vi "SectionA04_Week5_Stus_Subvi.vi"(9 "Frequency of Input (mHz)":dbl, 10 "Gain":dbl, 11 "Peak Voltage of Input":dbl) -> (3 "Array":dbl[][](array[numeric]))   [LabVIEW 2013]
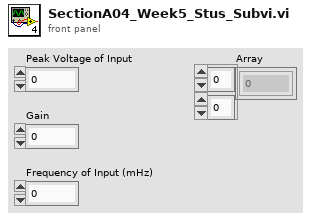
[diagram p1: front panel]
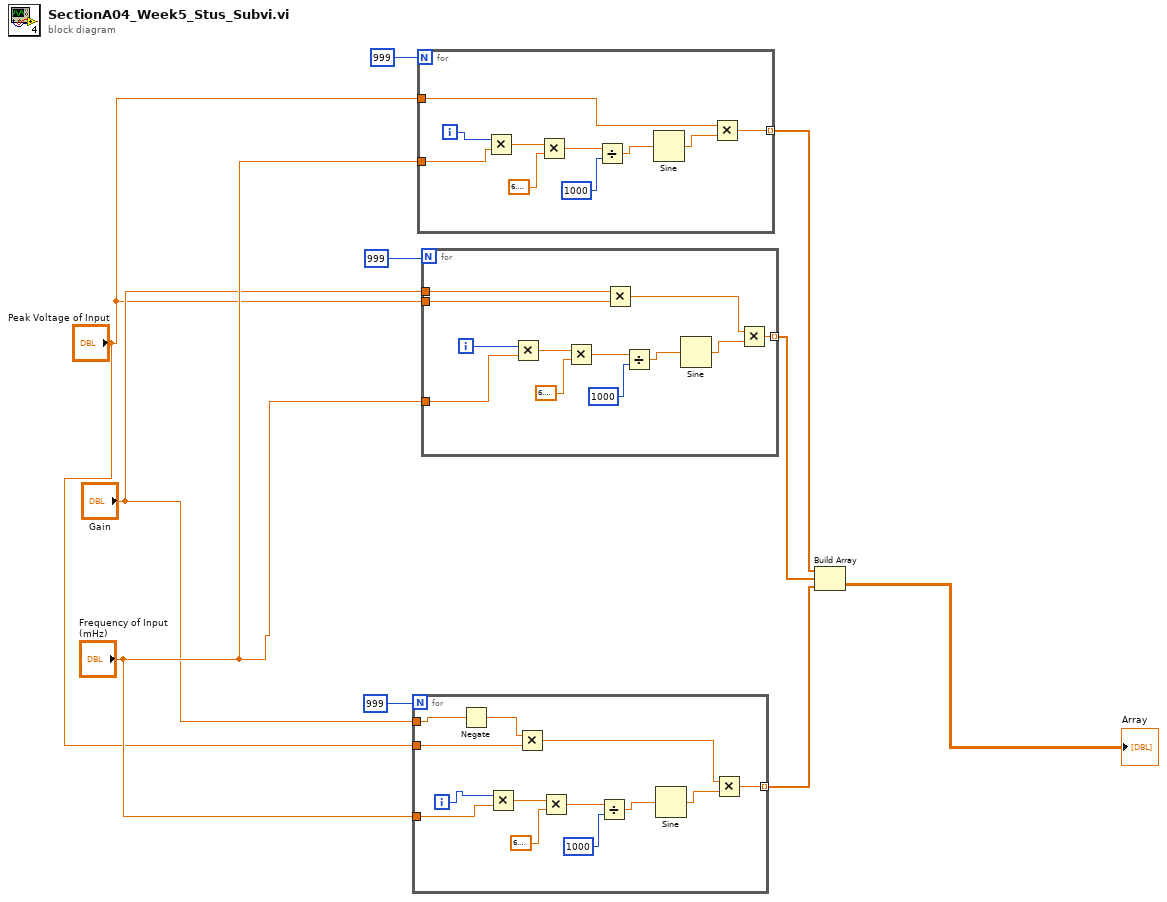
[diagram p0: block diagram]
diagram:
  n1 = for {
    N: 999 -> [_]
    tunnel: "Frequency of Input (mHz)" -> [w17]
    tunnel: "Gain" -> [w12]
    tunnel: "Peak Voltage of Input" -> [w15]
    tunnel: [w13] -> w9 mode=indexing
    i -> [w16]
    n2 = Negate(x=w12) -> (-x=w11:dbl)
    n3 = Multiply(x=w16, y=w17) -> (x*y=w23:dbl)
    n4 = Multiply(x=w11, y=w15) -> (x*y=w14:dbl)
    n5 = Multiply(x=w23, y=6.283185307179586) -> (x*y=w21:dbl)
    n6 = Divide(x=w21, y=1000) -> (x/y=w19:dbl)
    n7 = Sine(x=w19) -> (sin(x)=w18:dbl)
    n8 = Multiply(x=w14, y=w18) -> (x*y=w13:dbl)
  }
  n9 = for {
    N: 999 -> [_]
    tunnel: "Frequency of Input (mHz)" -> [w27]
    tunnel: [w25] -> w7 mode=indexing
    tunnel: "Peak Voltage of Input" -> [w24]
    i -> [w26]
    n10 = Multiply(x=w26, y=w27) -> (x*y=w28:dbl)
    n11 = Multiply(x=w28, y=6.283185307179586) -> (x*y=w30:dbl)
    n12 = Divide(x=w30, y=1000) -> (x/y=w32:dbl)
    n13 = Sine(x=w32) -> (sin(x)=w33:dbl)
    n14 = Multiply(x=w24, y=w33) -> (x*y=w25:dbl)
  }
  n15 = for {
    N: 999 -> [_]
    tunnel: "Frequency of Input (mHz)" -> [w37]
    tunnel: "Gain" -> [w36]
    tunnel: "Peak Voltage of Input" -> [w35]
    tunnel: [w34] -> w2 mode=indexing
    i -> [w38]
    n16 = Multiply(x=w38, y=w37) -> (x*y=w45:dbl)
    n17 = Multiply(x=w45, y=6.283185307179586) -> (x*y=w43:dbl)
    n18 = Multiply(x=w36, y=w35) -> (x*y=w39:dbl)
    n19 = Divide(x=w43, y=1000) -> (x/y=w41:dbl)
    n20 = Sine(x=w41) -> (sin(x)=w40:dbl)
    n21 = Multiply(x=w39, y=w40) -> (x*y=w34:dbl)
  }
  n22 = Build Array(w7, w2, w9) -> (→"Array":dbl[][])
